vi "FTW-Publisher-Listener.vi"(1 "keep most recent":i32=1, 2 "Timeout":i32=-1, 3 "FTW Endpoint":refnum<class "FTW-Endpoint.lvclass">, 4 "FTW Publisher":refnum<class "FTW-Publisher.lvclass">) -> ()   [LabVIEW 2015, in "FTW-Publisher.lvclass"]
uses:
  FTW-Publisher.lvclass
  Endpoint/FTW-Endpoint.lvclass
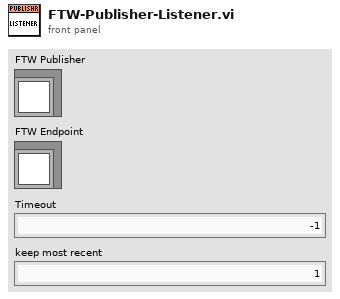
[diagram p1: front panel]
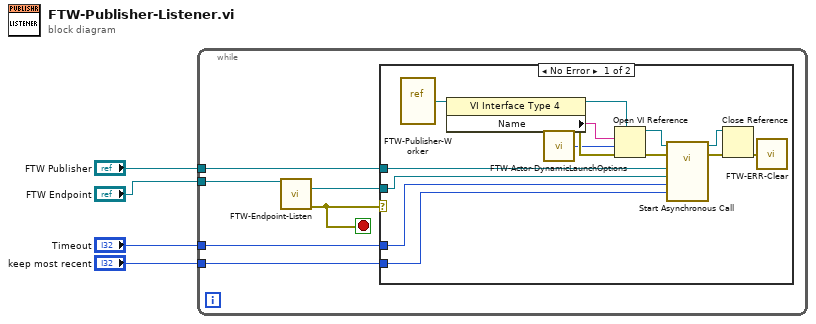
[diagram p0: block diagram]
diagram:
  n1 = while {
    tunnel: "FTW Publisher" -> [w6]
    tunnel: "Timeout" -> [w8]
    tunnel: "keep most recent" -> [w7]
    tunnel: "FTW Endpoint" -> [w5]
    stop <- w10 stop-if-true
    n2 = call-dynamic "FTW-Endpoint-Listen.vi"("FTW Endpoint"=w5) -> ("New Connection"=w9:refnum<class "FTW-Endpoint.lvclass">, "error out"=w10:errorcluster)  [unwired: 12 in, 1 out]
    n3 = case shown="No Error" w10 {
      tunnel: w6 -> [w11 _]
      tunnel: w9 -> [w14 _]
      tunnel: w8 -> [w13 _]
      tunnel: w7 -> [w12 _]
      frame No Error {
        n4 = vi-ref "FTW-Publisher-Worker.vi"() -> (w24:refnum<vi>)
        n5 = property class="VI Interface Type 4"(reference=w24) -> (reference out=w18:refnum<vi>, error out=w23:errorcluster, "Name"=w22:string)  [unwired: 1 in]
        n6 = call "FTW-Actor-DynamicLaunchOptions.vi"() -> ("Open VI Ref Options"=w21:i32)
        n7 = Open VI Reference(type specifier VI Refnum (for type only)=w18, vi path=w22, options=w21, error in (no error)=w23) -> (vi reference=w19:refnum<vi>, error out=w20:errorcluster)  [unwired: 2 in]
        n8 = call-by-ref "Start Asynchronous Call"(reference=w19, error in=w20, "keep most recent"=w12, "Timeout"=w13, "Endpoint"=w14, "Worker Pipes"=w11) -> (reference out=w15:refnum<vi>, error out=w17:errorcluster)  [unwired: 1 in]
        n9 = Close Reference(reference=w15, error in (no error)=w17) -> (error out=w16:errorcluster)
        n10 = call "FTW-ERR-Clear.vi"("error to snuff"=w16) -> ()  [unwired: 1 out]
      }
      frame Error {
      }
    }
  }
